vi "KB-DealWith Signal Picture.vi"(0 "Imaq1":T1, 1 "CCD1":string, 5 "Param List CCD":string[][](array[string])=[[";1650.000;1055.000;162.000;324.000;0.000;0.000;0;1;3;3;15.000;4;0;1;0;0;1;65280;255;16776960;16711680;", ";1645.000;1058.000;62.000;156.000;0.000;0.000;0;1;13;13;52.000;4;0;1;0;0;1;65280;255;16776960;16711680;", "Null", "Null", "Null", "Null", "Null", "Null", "Null", "Null"], [";1666.000;992.000;164.000;329.000;0.000;0.000;0;1;3;3;12.000;4;0;1;0;0;1;65280;255;16776960;16711680;", ";1644.000;989.000;75.000;150.000;0.000;0.000;0;2;13;13;52.000;4;0;1;0;0;1;65280;255;16776960;16711680;", "Null", "Null", "Null", "Null", "Null", "Null", "Null", "Null"], [";1641.000;1097.000;175.000;301.000;0.000;0.000;0;1;3;3;12.000;4;0;1;0;0;1;65280;255;16776960;16711680;", ";1637.000;1088.000;74.000;149.000;0.000;0.000;0;2;13;13;52.000;4;0;1;0;0;1;65280;255;16776960;16711680;", "Null", "Null", "Null", "Null", "Null", "Null", "Null", "Null"], [";1645.000;1085.000;198.000;330.000;0.000;0.000;0;1;3;3;12.000;4;0;1;0;0;1;65280;255;16776960;16711680;", ";1649.000;1092.000;69.000;146.000;0.000;0.000;0;2;13;13;52.000;4;0;1;0;0;1;65280;255;16776960;16711680;", "Null", "Null", "Null", "Null", "Null", "Null", "Null", "Null"], [";1646.000;1097.000;198.000;323.000;0.000;0.000;0;1;3;3;12.000;4;0;1;0;0;1;65280;255;16776960;16711680;", ";1647.000;1093.000;74.000;149.000;0.000;0.000;0;2;19;13;52.000;4;0;1;0;0;1;65280;255;16776960;16711680;", "Null", "Null", "Null", "Null", "Null", "Null", "Null", "Null"], [";1650.000;1035.000;192.000;317.000;0.000;0.000;0;1;3;3;12.000;4;0;1;0;0;1;65280;255;16776960;16711680;", ";1669.000;1059.000;33.000;161.000;0.000;0.000;0;2;19;13;52.000;4;0;1;0;0;1;65280;255;16776960;16711680;", "Null", "Null", "Null", "Null", "Null", "Null", "Null", "Null"], [";1549.000;1024.000;204.000;306.000;0.000;0.000;0;1;3;3;12.000;4;0;1;0;0;1;65280;255;16776960;16711680;", ";1546.000;1027.000;72.000;144.000;0.000;0.000;0;2;19;13;52.000;4;0;1;0;0;1;65280;255;16776960;16711680;", "Null", "Null", "Null", "Null", "Null", "Null", "Null", "Null"], [";1552.000;926.000;174.000;303.000;0.000;0.000;0;1;19;13;52.000;4;0;1;0;0;1;65280;255;16776960;16711680;", ";1553.000;934.000;72.000;145.000;0.000;0.000;0;2;19;13;52.000;4;0;1;0;0;1;65280;255;16776960;16711680;", "Null", "Null", "Null", "Null", "Null", "Null", "Null", "Null"], [";1546.000;954.000;166.000;315.000;0.000;0.000;0;1;3;3;12.000;4;0;1;0;0;1;65280;255;16776960;16711680;", ";1547.000;950.000;73.000;147.000;0.000;0.000;0;2;19;13;52.000;4;0;1;0;0;1;65280;255;16776960;16711680;", "Null", "Null", "Null", "Null", "Null", "Null", "Null", "Null"], [";1543.000;971.000;184.000;314.000;0.000;0.000;0;1;3;3;12.000;4;0;1;0;0;1;65280;255;16776960;16711680;", ";1547.000;972.000;76.000;152.000;0.000;0.000;0;2;19;13;52.000;4;0;1;0;0;1;65280;255;16776960;16711680;", "Null", "Null", "Null", "Null", "Null", "Null", "Null", "Null"], [";1552.000;1013.000;185.000;317.000;0.000;0.000;0;1;3;3;12.000;4;0;1;0;0;1;65280;255;16776960;16711680;", ";1549.000;1013.000;72.000;145.000;0.000;0.000;0;2;19;13;52.000;4;0;1;0;0;1;65280;255;16776960;16711680;", "Null", "Null", "Null", "Null", "Null", "Null", "Null", "Null"], [";1560.000;910.000;181.000;316.000;0.000;0.000;0;1;3;3;12.000;4;0;1;0;0;1;65280;255;16776960;16711680;", ";1562.000;918.000;70.000;140.000;0.000;0.000;0;1;19;13;52.000;4;0;1;0;0;1;65280;255;16776960;16711680;", "Null", "Null", "Null", "Null", "Null", "Null", "Null", "Null"], [";1330.000;923.000;139.000;279.000;0.000;0.000;0;2;21;13;15.000;4;0;1;0;0;1;65280;255;16776960;16711680;", ";1328.000;918.000;70.000;141.000;0.000;0.000;0;2;21;13;45.000;4;0;1;0;0;1;65280;255;16776960;16711680;", "Null", "Null", "Null", "Null", "Null", "Null", "Null", "Null"], [";1370.000;1170.000;162.000;278.000;0.000;0.000;0;2;21;13;15.000;4;0;1;0;0;1;65280;255;16776960;16711680;", ";1367.000;1164.000;71.000;143.000;0.000;0.000;0;2;19;13;15.000;4;0;1;0;0;1;65280;255;16776960;16711680;", "Null", "Null", "Null", "Null", "Null", "Null", "Null", "Null"], [";1660.000;1110.000;150.000;301.000;0.000;0.000;0;2;21;13;15.000;4;0;1;0;0;1;65280;255;16776960;16711680;", ";1662.000;1114.000;78.000;156.000;0.000;0.000;0;2;21;13;25.000;4;0;1;0;0;1;65280;255;16776960;16711680;", "Null", "Null", "Null", "Null", "Null", "Null", "Null", "Null"], [";1611.000;1132.000;156.000;273.000;0.000;0.000;0;2;21;13;45.000;4;0;1;0;0;1;65280;255;16776960;16711680;", ";1613.000;1132.000;72.000;145.000;0.000;0.000;0;2;21;13;15.000;4;0;1;0;0;1;65280;255;16776960;16711680;", "Null", "Null", "Null", "Null", "Null", "Null", "Null", "Null"], [";1591.000;1169.000;165.000;294.000;0.000;0.000;0;1;13;13;15.000;4;0;1;0;0;1;65280;255;16776960;16711680;", ";1625.000;1187.000;75.000;150.000;0.000;0.000;0;2;13;13;55.000;4;0;1;0;0;1;65280;255;16776960;16711680;", "Null", "Null", "Null", "Null", "Null", "Null", "Null", "Null"], [";1586.000;1193.000;179.000;359.000;0.000;0.000;0;1;13;13;35.000;4;0;1;0;0;1;65280;255;16776960;16711680;", ";1614.000;1212.000;75.000;150.000;0.000;0.000;0;2;13;13;55.000;4;0;1;0;0;1;65280;255;16776960;16711680;", "Null", "Null", "Null", "Null", "Null", "Null", "Null", "Null"], [";1676.000;1155.000;175.000;350.000;0.000;0.000;0;1;13;13;55.000;4;0;1;0;0;1;65280;255;16776960;16711680;", ";1670.000;1157.000;70.000;141.000;0.000;0.000;0;2;13;13;55.000;4;0;1;0;0;1;65280;255;16776960;16711680;", "Null", "Null", "Null", "Null", "Null", "Null", "Null", "Null"], [";1620.000;1151.000;188.000;377.000;0.000;0.000;0;1;13;13;55.000;4;0;1;0;0;1;65280;255;16776960;16711680;", ";1613.000;1143.000;81.000;150.000;0.000;0.000;0;2;13;13;55.000;4;0;1;0;0;1;65280;255;16776960;16711680;", "Null", "Null", "Null", "Null", "Null", "Null", "Null", "Null"], [";1592.000;1152.000;179.000;359.000;0.000;0.000;0;1;13;13;55.000;4;0;1;0;0;1;65280;255;16776960;16711680;", ";1577.000;1142.000;75.000;151.000;0.000;0.000;0;2;13;13;55.000;4;0;1;0;0;1;65280;255;16776960;16711680;", "Null", "Null", "Null", "Null", "Null", "Null", "Null", "Null"], [";1284.000;1016.000;459.000;919.000;0.000;0.000;0;1;13;13;15.000;4;0;1;0;0;1;65280;255;16776960;16711680;", ";1286.000;1055.000;239.000;466.000;0.000;0.000;0;2;13;13;55.000;4;0;1;0;0;1;65280;255;16776960;16711680;", "Null", "Null", "Null", "Null", "Null", "Null", "Null", "Null"], [";1600.000;1172.000;534.000;991.000;0.000;0.000;0;1;13;13;15.000;4;0;1;0;0;1;65280;255;16776960;16711680;", ";1604.000;1188.000;203.000;406.000;0.000;0.000;0;2;15;13;43.000;4;0;1;0;0;1;65280;255;16776960;16711680;", "Null", "Null", "Null", "Null", "Null", "Null", "Null", "Null"], [";1836.000;828.000;597.000;1195.000;0.000;0.000;0;1;15;13;13.000;4;0;1;0;0;1;65280;255;16776960;16711680;", ";1840.000;824.000;216.000;432.000;0.000;0.000;0;2;5;13;43.000;4;0;1;0;0;1;65280;255;16776960;16711680;", "Null", "Null", "Null", "Null", "Null", "Null", "Null", "Null"], [";1583.000;947.000;487.000;975.000;0.000;0.000;0;1;13;13;13.000;4;0;1;0;0;1;65280;255;16776960;16711680;", ";1583.000;941.000;211.000;397.000;0.000;0.000;0;2;5;13;43.000;4;0;1;0;0;1;65280;255;16776960;16711680;", "Null", "Null", "Null", "Null", "Null", "Null", "Null", "Null"], [";1841.000;926.000;497.000;995.000;0.000;0.000;0;1;13;13;13.000;4;0;1;0;0;1;65280;255;16776960;16711680;", ";1820.000;924.000;209.000;418.000;0.000;0.000;0;2;13;13;13.000;4;0;1;0;0;1;65280;255;16776960;16711680;", "Null", "Null", "Null", "Null", "Null", "Null", "Null", "Null"], [";1728.000;864.000;582.000;1165.000;0.000;0.000;0;1;13;13;13.000;4;0;1;0;0;1;65280;255;16776960;16711680;", ";1720.000;888.000;203.000;406.000;0.000;0.000;0;2;13;13;13.000;4;0;1;0;0;1;65280;255;16776960;16711680;", "Null", "Null", "Null", "Null", "Null", "Null", "Null", "Null"], [";1508.000;1012.000;497.000;878.000;0.000;0.000;0;1;13;13;13.000;4;0;1;0;0;1;65280;255;16776960;16711680;", ";1520.000;1008.000;206.000;413.000;0.000;0.000;0;2;13;13;13.000;4;0;1;0;0;1;65280;255;16776960;16711680;", "Null", "Null", "Null", "Null", "Null", "Null", "Null", "Null"], [";2110.000;860.000;450.000;901.000;0.000;0.000;0;1;13;13;13.000;4;0;1;0;0;1;65280;255;16776960;16711680;", ";2105.000;860.000;205.000;410.000;0.000;0.000;0;2;15;13;13.000;4;0;1;0;0;1;65280;255;16776960;16711680;", "Null", "Null", "Null", "Null", "Null", "Null", "Null", "Null"], [";1900.000;1200.000;491.000;983.000;0.000;0.000;0;1;15;13;13.000;4;0;1;0;0;1;65280;255;16776960;16711680;", ";1877.000;1223.000;205.000;411.000;0.000;0.000;0;2;19;13;55.000;4;0;1;0;0;1;65280;255;16776960;16711680;", "Null", "Null", "Null", "Null", "Null", "Null", "Null", "Null"], [";2850.000;740.000;530.000;933.000;0.000;0.000;0;1;13;13;15.000;4;0;1;0;0;1;65280;255;16776960;16711680;", ";2849.000;737.000;215.000;404.000;0.000;0.000;0;2;13;13;15.000;4;0;1;0;0;1;65280;255;16776960;16711680;", "Null", "Null", "Null", "Null", "Null", "Null", "Null", "Null"], ["Null", "Null", "Null", "Null", "Null", "Null", "Null", "Null", "Null", "Null"], ["Null", "Null", "Null", "Null", "Null", "Null", "Null", "Null", "Null", "Null"]], 7 "索引 (行)":i32, 11 "Color Select":string(combo)="白色", 12 "CCD2":string, 13 "error in":errorcluster) -> (6 "Image Out":T1, 8 "结果":string[](array[string]), 14 "error out":errorcluster, 15 "数组":sgl[](array[numeric]))   [LabVIEW 2015]
uses:
  <vilib>/vision/Image Controls.llb/IMAQ Image.ctl
panel:
  out "x/y":dbl
  out "毫秒计时值":u32
  out "路径":path
  out "数值":i32
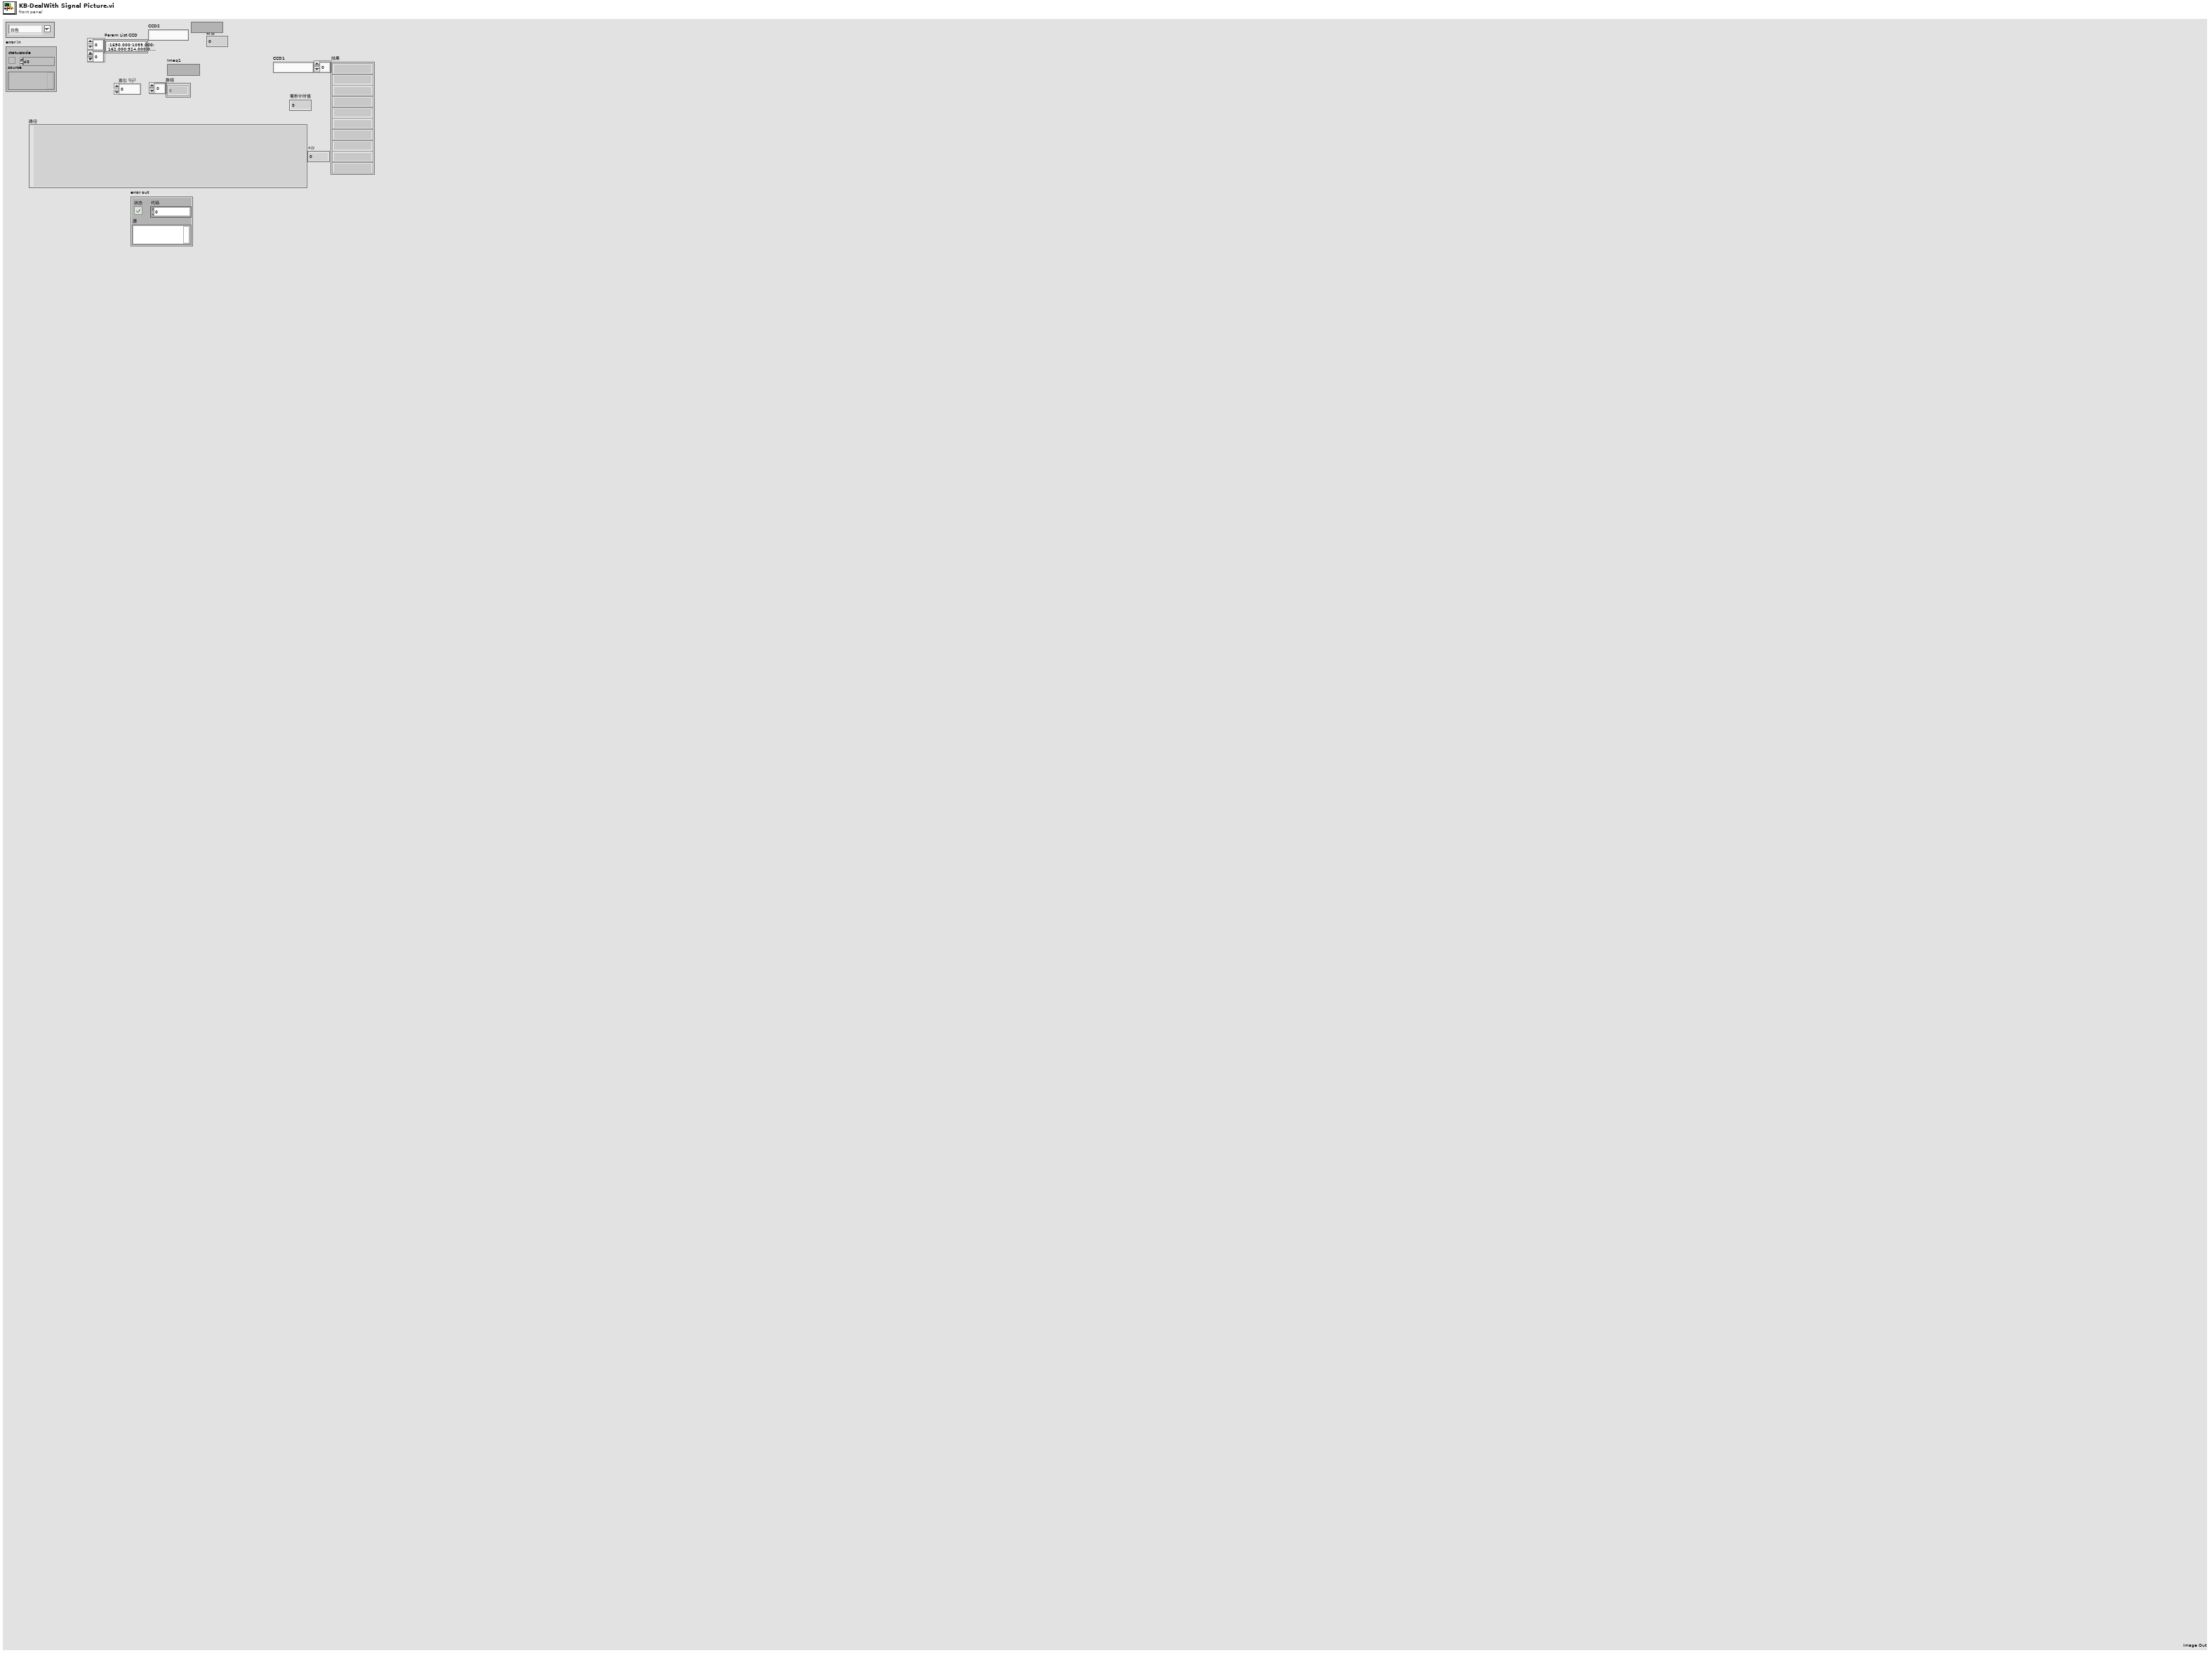
[diagram p1: front panel]
types:
  T1 = typedef "IMAQ Image.ctl" = refnum<image>
  T2 = typedef "Image Type" = u32
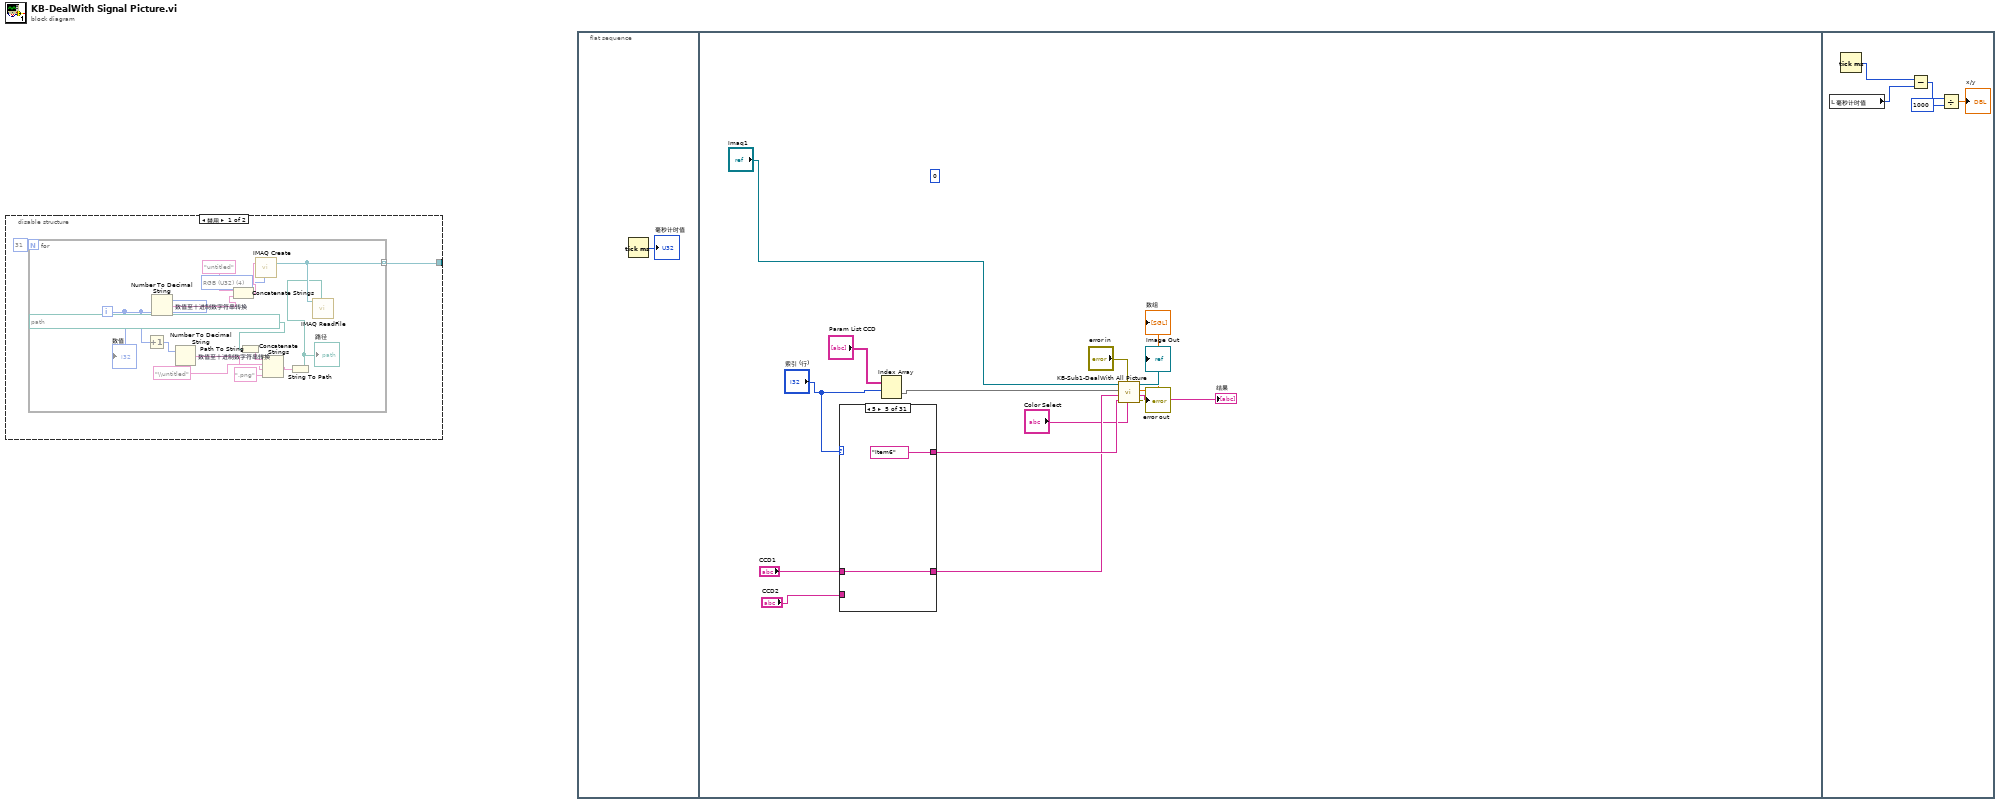
[diagram p0: block diagram]
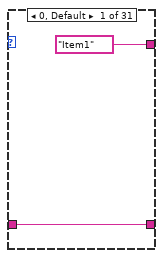
[diagram p2: hidden frame]
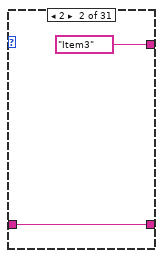
[diagram p3: hidden frame]
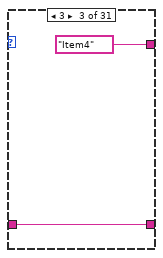
[diagram p4: hidden frame]
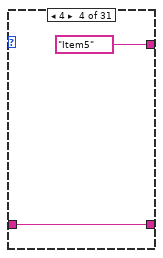
[diagram p5: hidden frame]
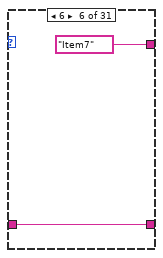
[diagram p6: hidden frame]
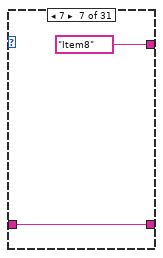
[diagram p7: hidden frame]
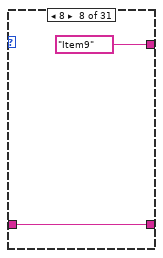
[diagram p8: hidden frame]
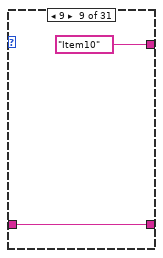
[diagram p9: hidden frame]
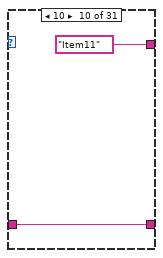
[diagram p10: hidden frame]
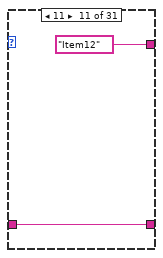
[diagram p11: hidden frame]
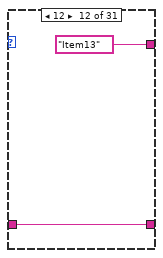
[diagram p12: hidden frame]
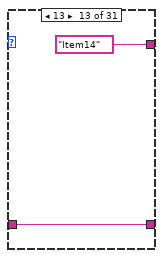
[diagram p13: hidden frame]
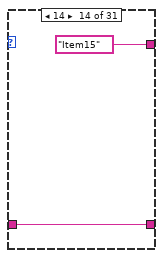
[diagram p14: hidden frame]
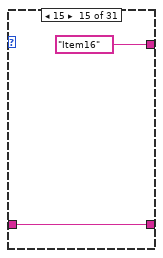
[diagram p15: hidden frame]
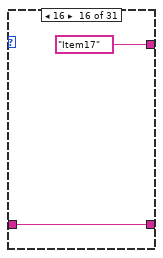
[diagram p16: hidden frame]
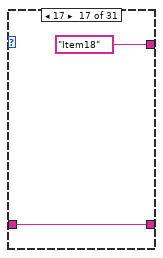
[diagram p17: hidden frame]
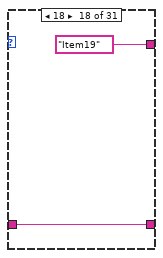
[diagram p18: hidden frame]
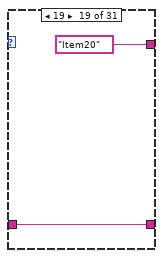
[diagram p19: hidden frame]
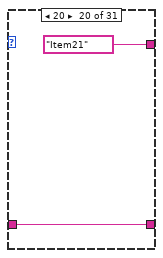
[diagram p20: hidden frame]
diagram:
  n1 = disable-structure shown="禁用" {
    disable-tunnel: [w1 _] -> _
    frame Disabled {
      n2 = for {
        N: 31 -> [_]
        tunnel: [w13] -> w1 mode=indexing
        i -> [w5]
        w14 = T2 4 items=["Grayscale (U8)", "Grayscale (I16)", "Grayscale (SGL)", "Complex (CSG)", "RGB (U32)", "HSL (U32)", "RGB (U64)", "Grayscale (U16)"] ("Image Type")
        n3 = Increment(x=w5) -> (x+1=w4:i32)
        n4 = Number To Decimal String "数值至十进制数字符串转换"(number=w5) -> (decimal integer string=w9:string)  [unwired: 1 in]
        n5 = Number To Decimal String "数值至十进制数字符串转换"(number=w4) -> (decimal integer string=w3:string)  [unwired: 1 in]
        n6 = Concatenate Strings("untitled" ("Image Name"), w9) -> (w15:string)
        n7 = Path To String(path=path "C:/Users/Administrator.PC-20160727FSNO/Desktop/新建文件夹" ("File Path")) -> (string=w11:string)
        n8 = call "IMAQ Create"("Image Name"=w15, "Image Type"=w14) -> ("New Image"=w13:T1)  [unwired: 3 in, 1 out]
        n9 = Concatenate Strings(w11, "\\untitled" ("字符串"), w3, ".png" ("字符串")) -> (w7:string)
        n10 = String To Path(string=w7) -> (path=w6:path)
        "路径" <- w6
        n11 = call "IMAQ ReadFile"("File Path"=w6, "Image"=w13) -> ()  [unwired: 5 in, 5 out]
        "数值" <- w5
      }
    }
    frame Enabled {
    }
  }
  n12 = flat-sequence {
    frame #0 {
      n13 = Tick Count (ms)() -> (millisecond timer value=→"毫秒计时值":u32)
    }
    frame #1 {
      (unwired) 0 ("索引")
      n14 = case shown="5" "索引 (行)" {
        tunnel: ["Item1" ("Row Select") "Item3" ("Row Select") "Item4" ("Row Select") "Item5" ("Row Select") "Item6" ("Row Select") "Item7" ("Row Select") "Item8" ("Row Select") "Item9" ("Row Select") "Item10" ("Row Select") "Item11" ("Row Select") "Item12" ("Row Select") "Item13" ("Row Select") "Item14" ("Row Select") "Item15" ("Row Select") "Item16" ("Row Select") "Item17" ("Row Select") "Item18" ("Row Select") "Item19" ("Row Select") "Item20" ("Row Select") "Item21" ("Row Select") "Item22" ("Row Select") "Item23" ("Row Select") "Item24" ("Row Select") "Item25" ("Row Select") "Item26" ("Row Select") "Item27" ("Row Select") "Item27" ("Row Select") "Item29" ("Row Select") "Item30" ("Row Select") "Item31" ("Row Select") "Item2" ("Row Select")] -> w27
        tunnel: "CCD1" -> [w32 w34 w36 w38 w40 w42 w44 w46 w48 w50 w52 w54 w56 w58 w60 w62 w64 w66 w68 w70 _ _ _ _ _ _ _ _ _ _ w92]
        tunnel: "CCD2" -> [_ _ _ _ _ _ _ _ _ _ _ _ _ _ _ _ _ _ _ _ w72 w74 w76 w78 w80 w82 w84 w86 w88 w90 _]
        tunnel: [w32 w34 w36 w38 w40 w42 w44 w46 w48 w50 w52 w54 w56 w58 w60 w62 w64 w66 w68 w70 w72 w74 w76 w78 w80 w82 w84 w86 w88 w90 w92] -> w24
        frame 0, Default {
        }
        frame 2 {
        }
        frame 3 {
        }
        frame 4 {
        }
        frame 5 {
        }
        frame 6 {
        }
        frame 7 {
        }
        frame 8 {
        }
        frame 9 {
        }
        frame 10 {
        }
        frame 11 {
        }
        frame 12 {
        }
        frame 13 {
        }
        frame 14 {
        }
        frame 15 {
        }
        frame 16 {
        }
        frame 17 {
        }
        frame 18 {
        }
        frame 19 {
        }
        frame 20 {
        }
        frame 21 {
        }
        frame 22 {
        }
        frame 23 {
        }
        frame 24 {
        }
        frame 25 {
        }
        frame 26 {
        }
        frame 27 {
        }
        frame 28 {
        }
        frame 29 {
        }
        frame 30 {
        }
        frame 1 {
        }
      }
      n15 = Index Array(array="Param List CCD", index (row)="索引 (行)") -> (element=w29:string[])  [unwired: 1 in]
      n16 = call "KB-Sub1-DealWith All Picture.vi"("Color Select"="Color Select", "error in"="error in", "Row Select"=w27, "相机分辨率"=w24, "参数"=w29, "Image  In"="Imaq1") -> ("error out"=→"error out":errorcluster, "结果"=→"结果":string[], "数组"=→"数组":sgl[], "Image Out"=→"Image Out":T1)  [unwired: 2 in]
    }
    frame #2 {
      n17 = local read "毫秒计时值"() -> (w97:u32)
      n18 = Tick Count (ms)() -> (millisecond timer value=w98:u32)
      n19 = Subtract(x=w98, y=w97) -> (x-y=w96:u32)
      n20 = Divide(x=w96, y=u32 1000) -> (x/y=→"x/y":dbl)
    }
  }
